vi "Import - Rx Packet.vi"(7 "Rx Packet":T1 {"targetPriority" min=-2 max=16 step=1; "targetProcessor" min=-2 max=16 step=1; "Endianness" items=["big-endian"=0, "little-endian"=2]}, 8 "error in (no error)":errorcluster, 11 "Device Item Ref in":T10 format="%.0x") -> (0 "error out":errorcluster)   [LabVIEW 2019, in "UDP-Custom-Device System Explorer.lvlib"]
uses:
  UDP-Custom-Device System Explorer.lvlib
  <vilib>/NI VeriStand/Custom Device API/Custom Device Item Ref.ctl
  Types/XML - New/ImpExp - Rx Packet Data.ctl
  <vilib>/NI VeriStand/Custom Device API/Custom Device Item Info.ctl
  Shared/Types/Shared - Channel Data Type.ctl
  Shared/Types/Shared - Buffered.PacketInfo.ctl
  Shared/Types/Shared - Pointer Encoding.ctl
  Shared/Types/Shared - Receive Buffer Options.ctl
  Shared/Types/Shared - Transmit Buffer Options.ctl
  Shared/Types/Shared - New Data Options.ctl
  Shared/Types/Shared - Thread Management.ctl
  <vilib>/NI VeriStand/Custom Device API/Custom Device Channel.ctl
  <vilib>/NI VeriStand/Custom Device API/Custom Device Channel Type.ctl
  Shared/Constants.vi
  Property Accessors/Shared Packet Accessors.lvlib
  Property Accessors/Rx Packet Accessors.lvlib
  <vilib>/NI VeriStand/Custom Device API/Custom Device API.lvlib
  Shared/UDP-Custom-Device Shared.lvlib
  Property Accessors/Rx Channel Accessors.lvlib
  Property Accessors/Rx Channel Section Accessors.lvlib
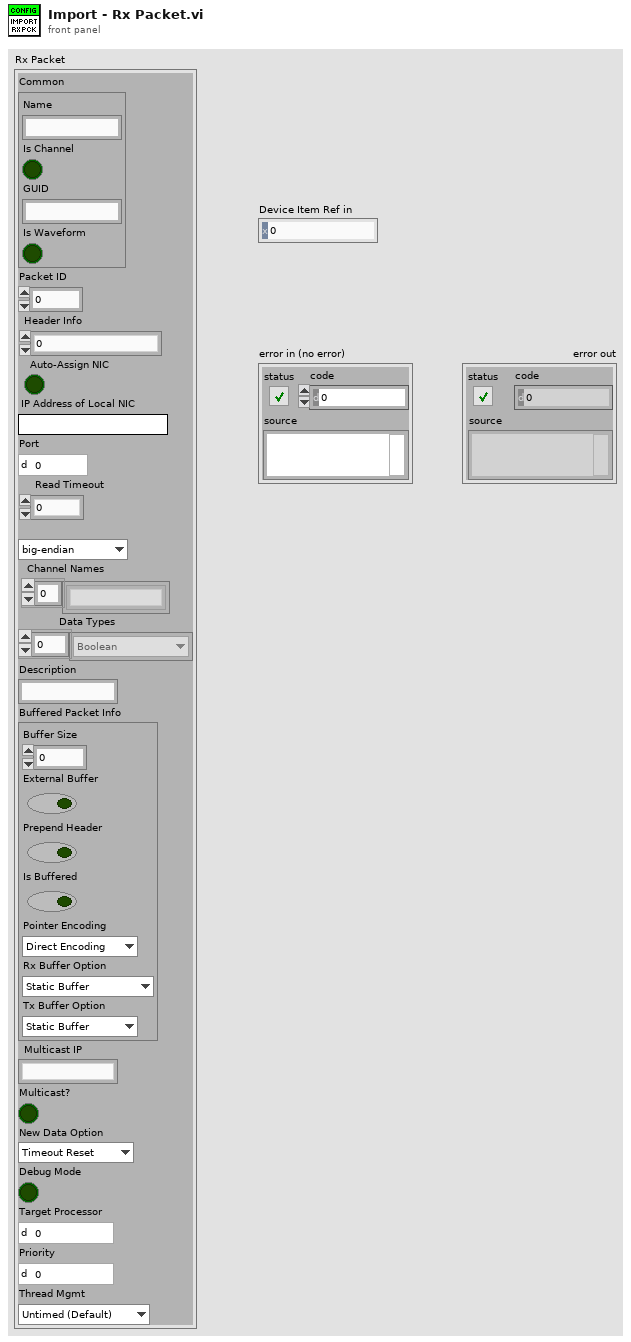
[diagram p1: front panel]
types:
  T1 = typedef "UDP-Custom-Device System Explorer.lvlib/ImpExp - Rx Packet Data.ctl" = cluster{"Common":T2, "Packet ID":i32, "Header Info":u32, "Auto-Assign NIC":bool, "IP Address of Local NIC":string, "Port":u16, "Read Timeout":i32, "Endianness":u16, "Channel Names":string[], "Data Types":T3[], "Description":string, "Buffered Packet Info":T4, "Multicast IP":string, "Multicast?":bool, "New Data Option":T8, "Debug Mode":bool, "targetProcessor":i8, "targetPriority":i16, "Thread Mgmt":T9}
  T2 = typedef "Custom Device API.lvlib/Custom Device Item Info.ctl" = cluster{"Name":string, "Is Channel":bool, "GUID":string, "Is Waveform":bool}
  T3 = typedef "UDP-Custom-Device Shared.lvlib/Shared - Channel Data Type.ctl" = enum16{"Boolean", "Single", "Double", "I8", "I16", "I32", "I64", "U8", "U16", "U32", "U64"}
  T4 = typedef "UDP-Custom-Device Shared.lvlib/Shared - Buffered.PacketInfo.ctl" = cluster{"Buffer Size":i32, "External Buffer":bool, "Prepend Header":bool, "Is Buffered":bool, "Pointer Encoding":T5, "Rx Buffer Option":T6, "Tx Buffer Option":T7}
  T5 = typedef "UDP-Custom-Device Shared.lvlib/Shared - Pointer Encoding.ctl" = enum16{"Direct Encoding", "Conversion Encoding"}
  T6 = typedef "UDP-Custom-Device Shared.lvlib/Shared - Receive Buffer Options.ctl" = enum16{"Static Buffer", "Circular Buffer", "Circular Buffer + Size", "Internal Cache", "Internal Cache + Size", "Ping Pong", "Ping Pong + Size"}
  T7 = typedef "UDP-Custom-Device Shared.lvlib/Shared - Transmit Buffer Options.ctl" = enum16{"Static Buffer", "FIFO Buffer", "FIFO Buffer + Port"}
  T8 = typedef "UDP-Custom-Device Shared.lvlib/Shared - New Data Options.ctl" = enum16{"Timeout Reset", "Counter"}
  T9 = typedef "UDP-Custom-Device Shared.lvlib/Shared - Thread Management.ctl" = enum16{"Untimed (Default)", "Timed (High Priority)"}
  T10 = typedef "Custom Device API.lvlib/Custom Device Item Ref.ctl" = u64
  T11 = typedef "Custom Device API.lvlib/Custom Device Channel.ctl" = cluster{"Type":T12, "Units":string, "Default Value":dbl, "Faultable":bool, "Scalable":bool}
  T12 = typedef "Custom Device API.lvlib/Custom Device Channel Type.ctl" = enum16{"Input", "Output"}
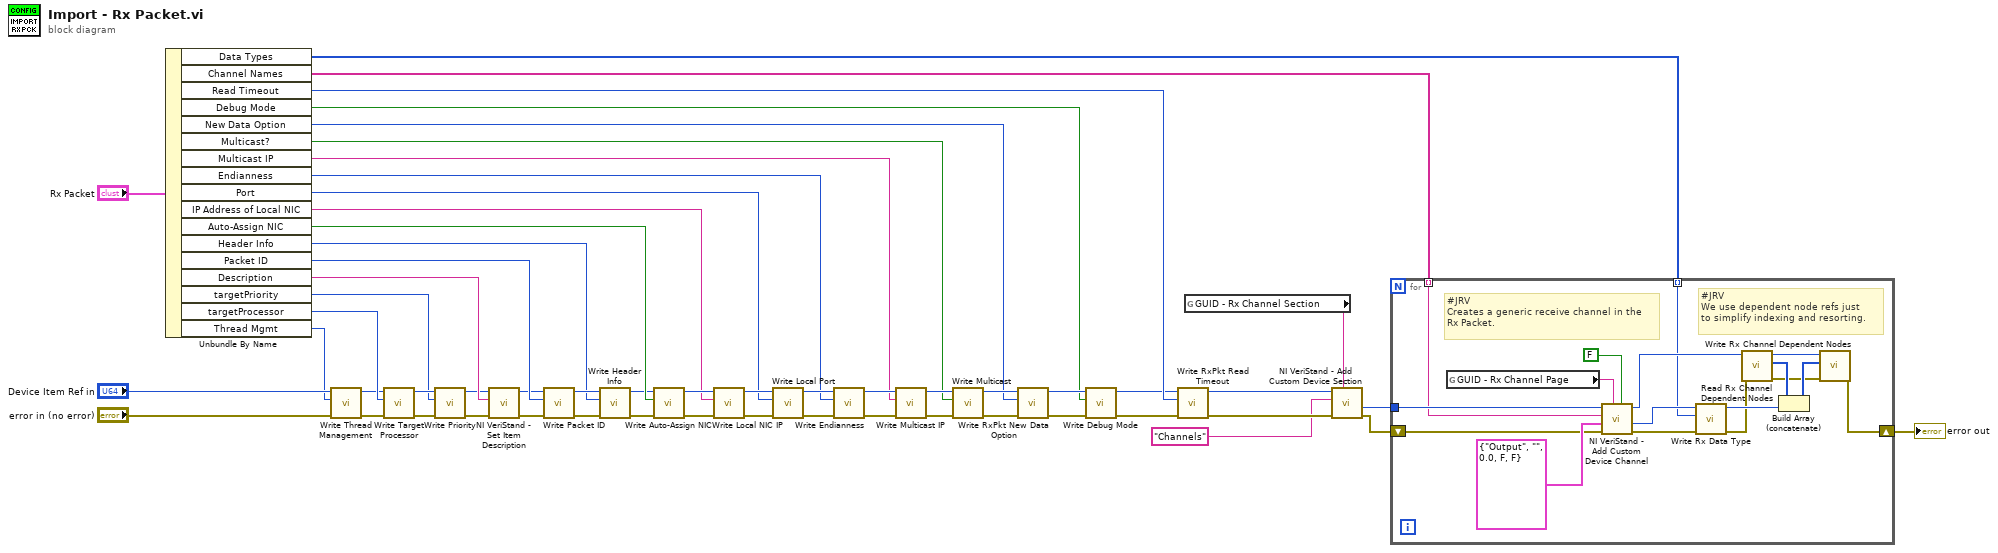
[diagram p0: block diagram]
diagram:
  n1 = Unbundle By Name("Rx Packet") -> ("Data Types"=w28:T3[], "Channel Names"=w27:string[], "Read Timeout"=w39:i32, "Debug Mode"=w12:bool, "New Data Option"=w17:T8, "Multicast?"=w20:bool, "Multicast IP"=w21:string, "Endianness"=w40:u16, "Port"=w43:u16, "IP Address of Local NIC"=w46:string, "Auto-Assign NIC"=w50:bool, "Header Info"=w51:u32, "Packet ID"=w54:i32, "Description"=w37:string, "targetPriority"=w7:i16, "targetProcessor"=w6:i8, "Thread Mgmt"=w1:T9)
  n2 = call "Write Thread Management.vi"("error in (no error)"="error in (no error)", "Thread Management"=w1, "Node Ptr"="Device Item Ref in") -> ("error out"=w2:errorcluster, "Node Ptr out"=w4:T10)  [unwired: 7 in]
  n3 = call "Write Target Processor.vi"("error in (no error)"=w2, "targetProcessor"=w6, "Node Ptr"=w4) -> ("error out"=w10:errorcluster, "Node Ptr out"=w11:T10)  [unwired: 7 in]
  n4 = call "Write Priority.vi"("error in (no error)"=w10, "targetPriority"=w7, "Node Ptr"=w11) -> ("error out"=w8:errorcluster, "Node Ptr out"=w9:T10)  [unwired: 7 in]
  n5 = call <vilib>:"NI VeriStand - Set Item Description.vi"("error in (no error)"=w8, "Description"=w37, "Item Ref in"=w9) -> ("error out"=w35:errorcluster, "Item Ref out"=w36:T10)  [unwired: 6 in, 1 out]
  n6 = call "Write Packet ID.vi"("error in (no error)"=w35, "Packet ID"=w54, "Node Ptr"=w36) -> ("error out"=w52:errorcluster, "Node Ptr out"=w53:T10)  [unwired: 7 in]
  n7 = call "Write Header Info.vi"("error in (no error)"=w52, "Header Info"=w51, "Node Ptr"=w53) -> ("error out"=w48:errorcluster, "Node Ptr out"=w49:T10)  [unwired: 7 in]
  n8 = call "Write Auto-Assign NIC.vi"("error in (no error)"=w48, "Auto-Assign NIC"=w50, "Node Ptr"=w49) -> ("error out"=w45:errorcluster, "Node Ptr out"=w47:T10)  [unwired: 7 in]
  n9 = call "Write Local NIC IP.vi"("error in (no error)"=w45, "IP Address of Local NIC"=w46, "Node Ptr"=w47) -> ("error out"=w42:errorcluster, "Node Ptr out"=w44:T10)  [unwired: 7 in]
  n10 = call "Write Local Port.vi"("error in (no error)"=w42, "Port"=w43, "Node Ptr"=w44) -> ("error out"=w38:errorcluster, "Node Ptr out"=w41:T10)  [unwired: 7 in]
  n11 = call "Write Endianness.vi"("error in (no error)"=w38, "Endianness"=w40, "Node Ptr"=w41) -> ("error out"=w23:errorcluster, "Node Ptr out"=w22:T10)  [unwired: 7 in]
  n12 = call "Write Multicast IP.vi"("error in (no error)"=w23, "Multicast IP Address"=w21, "Node Ptr"=w22) -> ("error out"=w25:errorcluster, "Node Ptr out"=w24:T10)  [unwired: 7 in]
  n13 = call "Write Multicast.vi"("error in (no error)"=w25, "Multicast"=w20, "Node Ptr"=w24) -> ("error out"=w18:errorcluster, "Node Ptr out"=w19:T10)  [unwired: 7 in]
  n14 = call "Write RxPkt New Data Option.vi"("error in (no error)"=w18, "New Data Option"=w17, "Node Ptr"=w19) -> ("error out"=w14:errorcluster, "Node Ptr out"=w16:T10)  [unwired: 7 in]
  n15 = call "Write Debug Mode.vi"("error in (no error)"=w14, "Debug Mode"=w12, "Node Ptr"=w16) -> ("error out"=w13:errorcluster, "Node Ptr out"=w15:T10)  [unwired: 7 in]
  n16 = call "Write RxPkt Read Timeout.vi"("error in (no error)"=w13, "Read Timeout"=w39, "Node Ptr"=w15) -> ("error out"=w33:errorcluster, "Node Ptr out"=w34:T10)  [unwired: 7 in]
  n17 = global read "Constants.vi" "GUID - Rx Channel Section"() -> (w31:string)
  n18 = call <vilib>:"NI VeriStand - Add Custom Device Section.vi"("GUID (Default Section)"=w31, "error in (no error)"=w33, "Section Name"="Channels", "Parent Ref in"=w34) -> ("error out"=w29:errorcluster, "Section Ptr"=w30:T10)  [unwired: 4 in, 2 out]
  n19 = for {
    tunnel: w30 -> [w60]
    tunnel: w28 -> [w58] mode=indexing
    tunnel: w27 -> [w57] mode=indexing
    shift-right: [w56] -> w26
    shift-left: w29 -> [w59]
    # "#JRV\nWe use dependent node refs just\nto simplify indexing and resorting."
    # "#JRV\nCreates a generic receive channel in the \nRx Packet."
    n20 = global read "Constants.vi" "GUID - Rx Channel Page"() -> (w72:string)
    n21 = call <vilib>:"NI VeriStand - Add Custom Device Channel.vi"("Highlight? (F)"=FALSE, "GUID (Default Channel)"=w72, "error in (no error)"=w59, "Channel"=T11 {"Type"=enum."Output", "Units"="", "Default Value"=0.0, "Faultable"=FALSE, "Scalable"=FALSE}, "Channel Name"=w57, "Parent Ref in"=w60) -> ("error out"=w68:errorcluster, "Channel Ref"=w69:T10, "Parent Ref out"=w66:T10)  [unwired: 2 in, 1 out]
    n22 = call "Write Rx Data Type.vi"("error in (no error)"=w68, "Data Type"=w58, "Node Ptr"=w69) -> ("error out"=w65:errorcluster, "Node Ptr out"=w67:T10)  [unwired: 7 in]
    n23 = call "Read Rx Channel Dependent Nodes.vi"("error in (no error)"=w65, "Node Ptr"=w66) -> ("error out"=w61:errorcluster, "Dependent Node Refs"=w63:T10[], "Node Ptr out"=w64:T10)  [unwired: 7 in]
    n24 = Build Array (concatenate)(w63, w67) -> (w62:T10[])
    n25 = call "Write Rx Channel Dependent Nodes.vi"("error in (no error)"=w61, "Dependent Node Refs"=w62, "Node Ptr"=w64) -> ("error out"=w56:errorcluster)  [unwired: 7 in, 1 out]
  }
  "error out" <- w26
